vi "Perform Action.vi"(8 "error in (no error)":errorcluster, 10 "Message in":refnum<class "Message.lvclass">, 11 "OOQMH in":refnum<class "OOQMH.lvclass">) -> (0 "error out":errorcluster, 3 "OOQMH out":refnum<class "OOQMH.lvclass">)   [LabVIEW 2024, in "OOQMH.lvlib" / "OOQMH.lvclass"]
uses:
  OOQMH.lvclass
  Message/Message.lvclass
  OOQMH.lvclass/OOQMH.ctl
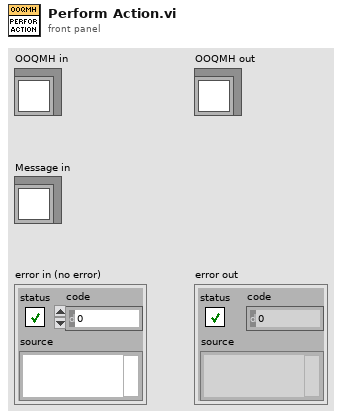
[diagram p1: front panel]
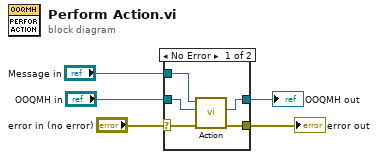
[diagram p0: block diagram]
diagram:
  n1 = case shown="No Error" "error in (no error)" {
    selector: "error in (no error)" -> [w7 w12]
    tunnel: [w6 w12] -> w4
    tunnel: [w9 w11] -> w2
    tunnel: "OOQMH in" -> [w10 w11]
    tunnel: "Message in" -> [w8 _]
    frame No Error {
      n2 = call-dynamic "Action.vi"("error in (no error)"=w7, "OOQMH in"=w10, "Message in"=w8) -> ("error out"=w6:errorcluster, "OOQMH out"=w9:refnum<class "OOQMH.lvclass">)  [unwired: 6 in, 1 out]
    }
    frame Error {
    }
  }
  "error out" <- w4
  "OOQMH out" <- w2
